vi "2023TestBegin.vi"   [LabVIEW 2020]
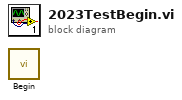
[diagram p0: block diagram]
diagram:
  n1 = call "Begin.vi"() -> ()  [unwired: 11 in, 1 out]
